vi "FL_Calculate_phi_theta_etc_3.vi"(0 "Input cluster of data":T1, 1 "SB size":u8, 2 "Bridge swap":bool, 3 "Use alternative magnets orientation":bool, 4 "Twisted neck":bool) -> (5 "Animal coordinates":T2)   [LabVIEW 2018, in "Tracker.lvlib"]
uses:
  Tracker.lvlib
  Controls/CTL_Animal_Coordinates_and_Speed.ctl
  Controls/CTL_Cage_Coords.ctl
  <vilib>/ptbypt/NI_PtbyPt.lvlib
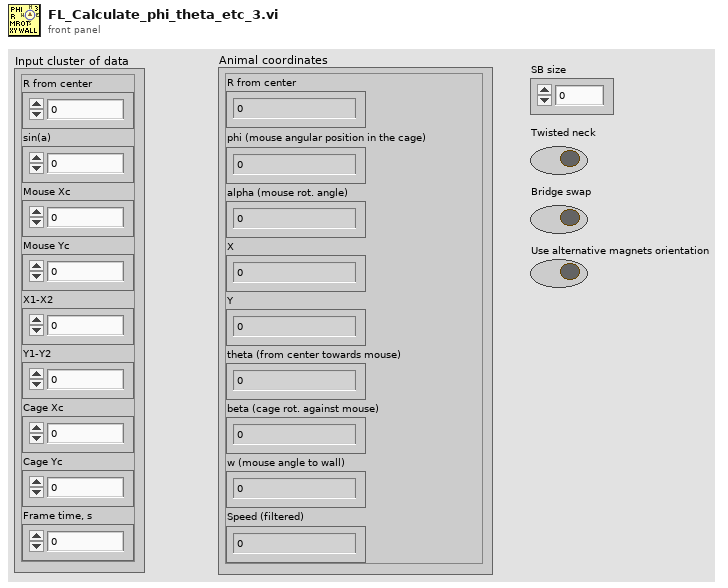
[diagram p1: front panel]
types:
  T1 = typedef "Tracker.lvlib/CTL_Cage_Coords.ctl" = cluster{"R from center":dbl, "sin(a)":dbl, "Mouse Xc":dbl, "Mouse Yc":dbl, "X1-X2":dbl, "Y1-Y2":dbl, "Cage Xc":dbl, "Cage Yc":dbl, "Frame time, s":dbl}
  T2 = typedef "Tracker.lvlib/CTL_Animal_Coordinates_and_Speed.ctl" = cluster{"R from center":dbl, "phi (mouse angular position in the cage)":dbl, "alpha (mouse rot. angle)":sgl, "X":dbl, "Y":dbl, "theta (from center towards mouse)":dbl, "beta (cage rot. against mouse)":sgl, "w (mouse angle to wall)":dbl, "Speed (filtered)":dbl}
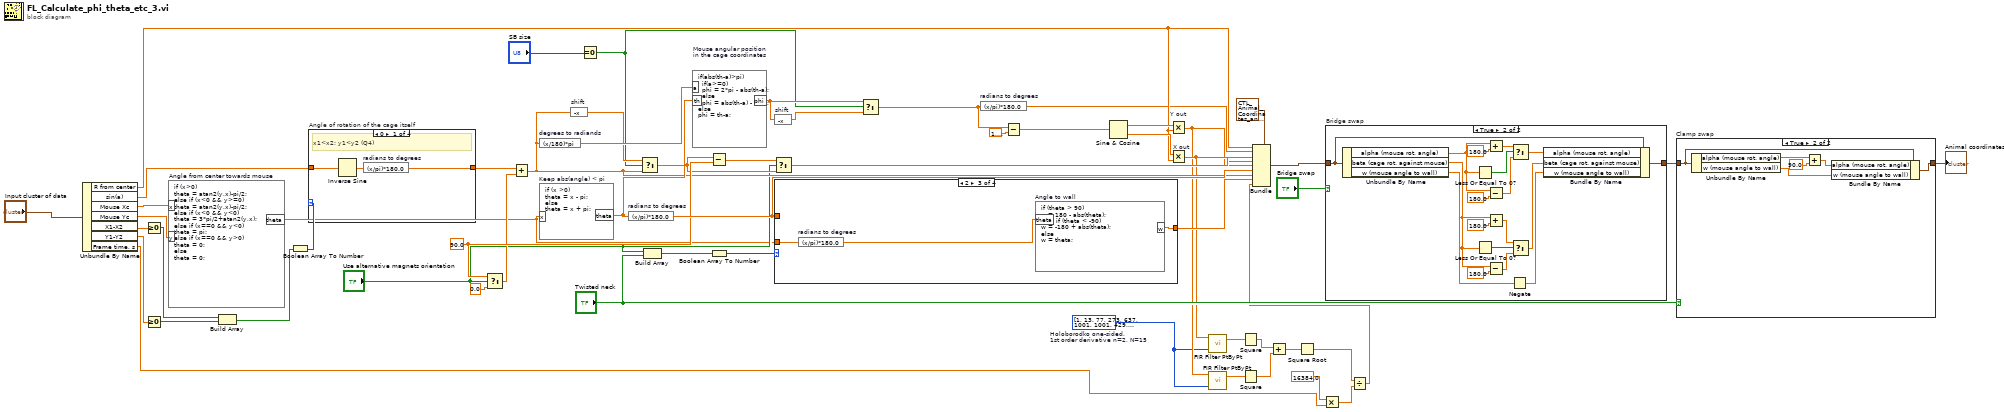
[diagram p0: block diagram]
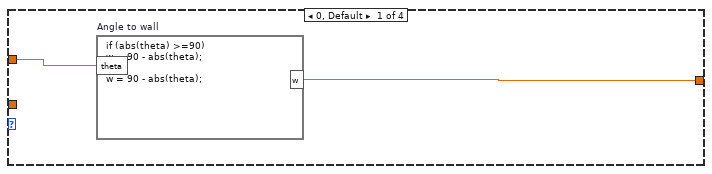
[diagram p3: hidden frame]
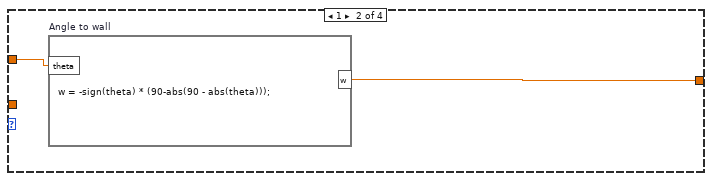
[diagram p4: hidden frame]
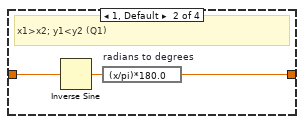
[diagram p7: hidden frame]
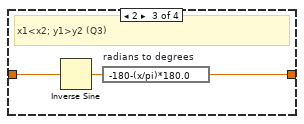
[diagram p8: hidden frame]
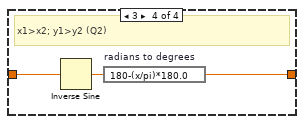
[diagram p9: hidden frame]
diagram:
  w11 = i32[] [1, 13, 77, 273, 637, 1001, 1001, 429, -429, -1001, -1001, -637, -273, -77, -13, -1]  # Holoborodko one-sided, 1st order derivative n=2, N=15
  w31 = 90.0 ("y")
  n1 = Unbundle By Name("Input cluster of data") -> ("R from center"=w40:dbl, "sin(a)"=w45:dbl, "Mouse Xc"=w44:dbl, "Mouse Yc"=w43:dbl, "X1-X2"=w42:dbl, "Y1-Y2"=w41:dbl, "Frame time, s"=w5:dbl)
  n2 = Greater Or Equal To 0?(x=w42) -> (x >= 0?=w57:bool)
  n3 = Greater Or Equal To 0?(x=w41) -> (x >= 0?=w56:bool)
  n4 = formula code="if (x>0)\ntheta = atan2(y,x)-pi/2;\nelse if (x<0 && y>=0)\ntheta = atan2(y,x)-pi/2;\nelse if (x<0 && y<0)\ntheta = 3*pi/2+atan2(y,x);\nelse if (x==0 && y<0)\ntheta = pi;\nelse if (x==0 && y>0)\ntheta = 0;\nelse\ntheta = 0;" "Angle from center towards mouse"("x"=w44, "y"=w43) -> ("theta"=w16:dbl)
  n5 = Build Array(w57, w56) -> (w55:bool[])
  n6 = Boolean Array To Number(Boolean array=w55) -> (number=w54:u32)
  n7 = case "Angle of rotation of the cage itself" shown="0" w54 {
    tunnel: w45 -> [w59 w62 w65 w68]
    tunnel: [w58 w61 w64 w67] -> w34
    frame 0 {
      # "x1<x2; y1<y2 (Q4)"
      n8 = Inverse Sine(1:w59) -> (0:w60:dbl)
      n9 = expression code="(x/pi)*180.0" "radians to degrees"(w60) -> (w58:dbl)
    }
    frame 1, Default {
      # "x1>x2; y1<y2 (Q1)"
      n10 = Inverse Sine(1:w62) -> (0:w63:dbl)
      n11 = expression code="(x/pi)*180.0" "radians to degrees"(w63) -> (w61:dbl)
    }
    frame 2 {
      # "x1<x2; y1>y2 (Q3)"
      n12 = Inverse Sine(1:w65) -> (0:w66:dbl)
      n13 = expression code="-180-(x/pi)*180.0" "radians to degrees"(w66) -> (w64:dbl)
    }
    frame 3 {
      # "x1>x2; y1>y2 (Q2)"
      n14 = Inverse Sine(1:w68) -> (0:w69:dbl)
      n15 = expression code="180-(x/pi)*180.0" "radians to degrees"(w69) -> (w67:dbl)
    }
  }
  n16 = Select(t=w31, s="Use alternative magnets orientation", f=0.0) -> (s? t:f=w30:dbl)
  n17 = Add(x=w34, y=w30) -> (x+y=w28:dbl)
  n18 = expression code="(x/180)*pi" "degrees to radiands"(w28) -> (w50:dbl)
  n19 = formula code="if (x >0)\ntheta = x - pi;\nelse\ntheta = x + pi;" "Keep abs(angle) < pi"("x"=w16) -> ("theta"=w51:dbl)
  n20 = expression code="-x" "shift"(w28) -> (w27:dbl)
  n21 = Equal To 0?(x="SB size") -> (x = 0?=w14:bool)
  n22 = expression code="(x/pi)*180.0" "radians to degrees"(w51) -> (w47:dbl)
  n23 = Select(t=w27, s=w14, f=w28) -> (s? t:f=w29:dbl)
  n24 = Build Array("Use alternative magnets orientation", "Twisted neck") -> (w18:bool[])
  n25 = formula code="if(abs(th-a)>pi)\n  if(a>=0)\n  phi = 2*pi - abs(th-a);\n  else\n  phi = abs(th-a) - 2*pi;\nelse\nphi = th-a;" "Mouse angular position in the cage coordinates"("th"=w51, "a"=w50) -> ("phi"=w25:dbl)
  n26 = Subtract(x=w29, y=w31) -> (x-y=w32:dbl)
  n27 = Boolean Array To Number(Boolean array=w18) -> (number=w17:u32)
  n28 = Select(t=w32, s="Use alternative magnets orientation", f=w29) -> (s? t:f=w33:dbl)
  n29 = expression code="-x" "shift"(w25) -> (w24:dbl)
  n30 = case shown="2" w17 {
    tunnel: w47 -> [w71 w73 _ w77]
    tunnel: [w70 w72 w76 w77] -> w21
    tunnel: w16 -> [_ _ w75 _]
    frame 0, Default {
      n31 = formula code="if (abs(theta) >=90)\nw = 90 - abs(theta);\nelse\nw = 90 - abs(theta);" "Angle to wall"("theta"=w71) -> ("w"=w70:dbl)
    }
    frame 1 {
      n32 = formula code="w = -sign(theta) * (90-abs(90 - abs(theta)));" "Angle to wall"("theta"=w73) -> ("w"=w72:dbl)
    }
    frame 2 {
      n33 = expression code="(x/pi)*180.0" "radians to degrees"(w75) -> (w74:dbl)
      n34 = formula code="if (theta > 90)\nw = 180 - abs(theta);\nelse if (theta < -90)\nw = -180 + abs(theta);\nelse\nw = theta;" "Angle to wall"("theta"=w74) -> ("w"=w76:dbl)
    }
    frame 3 {
    }
  }
  n35 = Select(t=w25, s=w14, f=w24) -> (s? t:f=w26:dbl)
  n36 = expression code="(x/pi)*180.0" "radians to degrees"(w26) -> (w39:dbl)
  n37 = Subtract(x=w26, y=1.5707963267948966) -> (x-y=w49:dbl)
  n38 = Sine & Cosine(0:w49) -> (1:w52:dbl, 2:w53:dbl)
  n39 = Multiply "Y out"(x=w52, y=w40) -> (x*y=w12:dbl)
  n40 = Multiply "X out"(x=w53, y=w40) -> (x*y=w13:dbl)
  n41 = call <vilib>:"FIR Filter PtByPt.vi"("Forward Coefficients"=w11, "x"=w13) -> ("Filtered x"=w10:dbl)  [unwired: 2 in, 1 out]
  n42 = call <vilib>:"FIR Filter PtByPt.vi"("Forward Coefficients"=w11, "x"=w12) -> ("Filtered x"=w9:dbl)  [unwired: 2 in, 1 out]
  n43 = Square(x=w10) -> (x^2=w8:dbl)
  n44 = Square(x=w9) -> (x^2=w7:dbl)
  n45 = Add(x=w8, y=w7) -> (x+y=w6:dbl)
  n46 = Square Root(x=w6) -> (sqrt(x)=w2:dbl)
  n47 = Multiply(x=16384.0 ("y"), y=w5) -> (x*y=w1:dbl)
  n48 = Divide(x=w2, y=w1) -> (x/y=w4:dbl)
  n49 = Bundle(cluster=T2 {"R from center"=0.0, "phi (mouse angular position in the cage)"=0.0, "alpha (mouse rot. angle)"=0.0, "X"=0.0, "Y"=0.0, "theta (from center towards mouse)"=0.0, "beta (cage rot. against mouse)"=0.0, "w (mouse angle to wall)"=0.0, "Speed (filtered)"=0.0} ("Output data cluster 2"), "R from center"=w40, "phi (mouse angular position in the cage)"=w39, "alpha (mouse rot. angle)"=w33, "X"=w13, "Y"=w12, "theta (from center towards mouse)"=w47, "beta (cage rot. against mouse)"=w28, "w (mouse angle to wall)"=w21, "Speed (filtered)"=w4) -> (w36:T2)
  n50 = case "Bridge swap" shown="True" "Bridge swap" {
    tunnel: [w78 w90] -> w23
    tunnel: w36 -> [w78 w91]
    frame False {
    }
    frame True {
      n51 = Unbundle By Name(w91) -> ("alpha (mouse rot. angle)"=w89:sgl, "beta (cage rot. against mouse)"=w82:sgl, "w (mouse angle to wall)"=w80:dbl)
      n52 = Less Or Equal To 0?(x=w89) -> (x <= 0?=w96:bool)
      n53 = Less Or Equal To 0?(x=w82) -> (x <= 0?=w83:bool)
      n54 = Add(x=w89, y=sgl 180.0) -> (x+y=w93:sgl)
      n55 = Subtract(x=w89, y=sgl 180.0) -> (x-y=w95:sgl)
      n56 = Add(x=w82, y=sgl 180.0) -> (x+y=w86:sgl)
      n57 = Subtract(x=w82, y=sgl 180.0) -> (x-y=w84:sgl)
      n58 = Negate(x=w80) -> (-x=w79:dbl)
      n59 = Select(t=w93, s=w96, f=w95) -> (s? t:f=w88:sgl)
      n60 = Select(t=w86, s=w83, f=w84) -> (s? t:f=w81:sgl)
      n61 = Bundle By Name(cluster=w91, "alpha (mouse rot. angle)"=w88, "beta (cage rot. against mouse)"=w81, "w (mouse angle to wall)"=w79) -> (w90:T2)
    }
  }
  n62 = case "Clamp swap" shown="True" "Twisted neck" {
    tunnel: [w97 w101] -> w22
    tunnel: w23 -> [w97 w102]
    frame False {
    }
    frame True {
      n63 = Unbundle By Name(w102) -> ("alpha (mouse rot. angle)"=w100:sgl, "w (mouse angle to wall)"=w99:dbl)
      n64 = Add(x=w100, y=sgl 90.0) -> (x+y=w98:sgl)
      n65 = Bundle By Name(cluster=w102, "alpha (mouse rot. angle)"=w98, "w (mouse angle to wall)"=w99) -> (w101:T2)
    }
  }
  "Animal coordinates" <- w22
